vi "Read Element of Exp Groups.vi"(8 "error in (no error)":errorcluster, 10 "Group #":i32=-1, 11 "Control-Client in":refnum<class "Control-Client.lvclass">) -> (0 "error out":errorcluster, 2 "Experiments_group.lvclass":refnum<class "Experiments_group.lvclass">, 3 "Control-Client out":refnum<class "Control-Client.lvclass">)   [LabVIEW 2015, in "Control-Client.lvclass"]
uses:
  Control-Client.lvclass
  Experiments/Experiments_group.lvclass
  Control-Client.lvclass/Control-Client.ctl
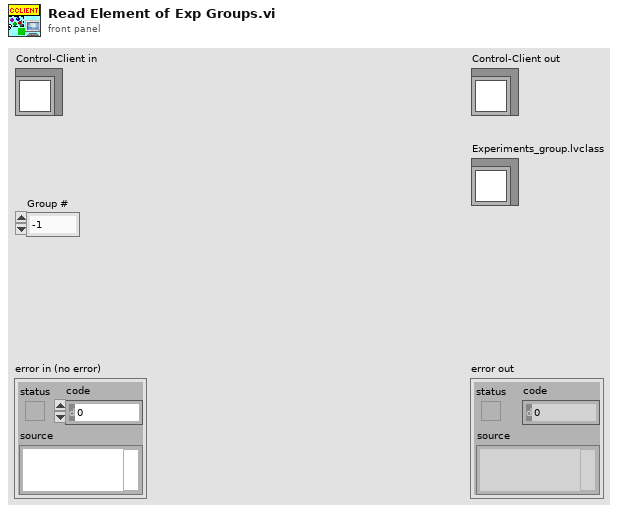
[diagram p1: front panel]
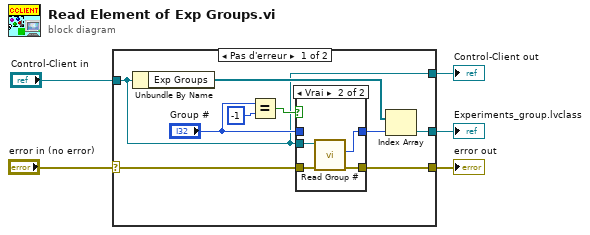
[diagram p0: block diagram]
diagram:
  n1 = case shown="Pas d'erreur" "error in (no error)" {
    selector: "error in (no error)" -> [w7 w21]
    tunnel: [w6 w21] -> w4
    tunnel: [w8 w22] -> w2
    tunnel: "Control-Client in" -> [w8 w22]
    tunnel: [w13 _] -> w1
    frame No Error {
      n2 = Unbundle By Name(w8) -> ("Exp Groups"=w14:refnum<class "Experiments_group.lvclass">[])
      n3 = Equal?(x="Group #", y=-1) -> (x = y?=w11:bool)
      n4 = case shown="Vrai" w11 {
        tunnel: [w16 w17] -> w10
        tunnel: "Group #" -> [w16 _]
        tunnel: w8 -> [_ w20]
        tunnel: w7 -> [w15 w19]
        tunnel: [w15 w18] -> w6
        frame False {
        }
        frame True {
          n5 = call "Read Group #.vi"("error in (no error)"=w19, "Control-Client in"=w20) -> ("error out"=w18:errorcluster, "Group #"=w17:i32)  [unwired: 7 in, 1 out]
        }
      }
      n6 = Index Array(array=w14, index=w10) -> (element=w13:refnum<class "Experiments_group.lvclass">)
    }
    frame Error {
    }
  }
  "error out" <- w4
  "Control-Client out" <- w2
  "Experiments_group.lvclass" <- w1
